vi "Update Parameter.vi"(7 "Action":enum16{"Increase", "Decrease"}(ring)=enum."Decrease", 10 "Modifier":i16, 11 "Parameter":i16) -> (3 "New Value":i16)   [LabVIEW 2026]
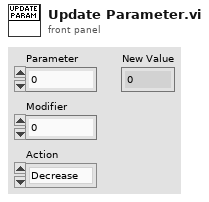
[diagram p1: front panel]
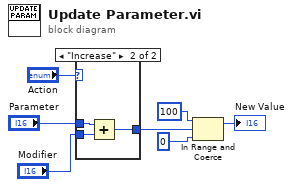
[diagram p0: block diagram]
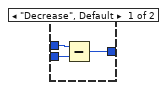
[diagram p2: hidden frame]
diagram:
  n1 = case shown="\"Increase\"" "Action" {
    tunnel: "Parameter" -> [w10 w13]
    tunnel: [w8 w12] -> w5
    tunnel: "Modifier" -> [w9 w11]
    frame "Decrease", Default {
      n2 = Subtract(x=w10, y=w9) -> (x-y=w8:i16)
    }
    frame "Increase" {
      n3 = Add(x=w13, y=w11) -> (x+y=w12:i16)
    }
  }
  n4 = In Range and Coerce(upper limit=i16 100, x=w5, lower limit=i16 0) -> (coerced(x)=→"New Value":i16)  [unwired: 1 out]
